vi "Cleanup.vi"(8 "error in":errorcluster, 11 "Refnum In":refnum<vi>) -> (0 "error out":errorcluster)   [LabVIEW 2020, in "FirmataClient.lvlib"]
doc: "Cleanup the library references, data and the actively selected transport (i.e. serial comport)"
uses:
  FirmataClient.lvlib
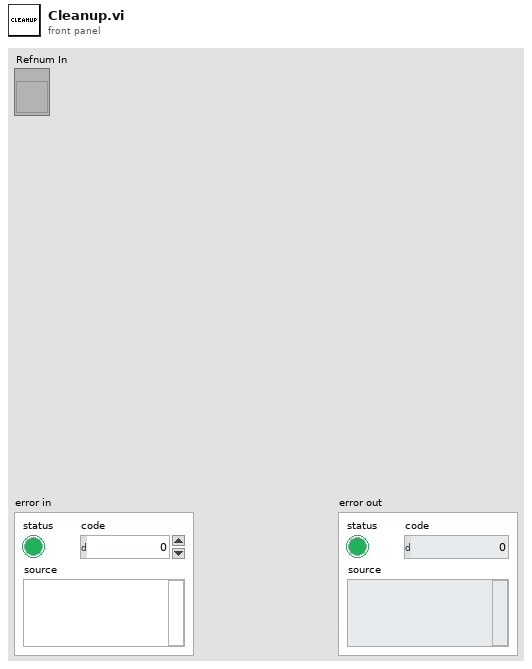
[diagram p1: front panel]
types:
  T1 = typedef "FirmataClient.lvlib/Parameters.ctl" = cluster{"Transport Parameters":T2, "Board Capabilities":map{i32, T4}}
  T2 = typedef "FirmataClient.lvlib/TransportParameters.ctl" = cluster{"Serial Communication":cluster{"Comport":refnum<visa-resource-name>, "No Response Timeout Ms":u32, "Response Complete Timeout Ms":u32, "Max Rx Length":u32, "Baud Rate":u32}, "Selected Transport":T3, "Initializer File Path":path, "Cleaner File Path":path, "Transporter File Path":path}
  T3 = typedef "FirmataClient.lvlib/SupportedTransports.ctl" = enum16{"Serial Communication Port"}
  T4 = typedef "FirmataClient.lvlib/FirmataPinCapabilitiesAndAnalogMapping.ctl" = cluster{"Supported Modes":T5[], "Analog Channel":u8, "Pin Name":string}
  T5 = typedef "FirmataClient.lvlib/FirmataPinCapability.ctl" = cluster{"PinMode":T6, "Resolution":u8}
  T6 = typedef "FirmataClient.lvlib/FirmataPinModes.ctl" = enum16{"DigitalInput", "DigitalOutput", "AnalogInput", "PWM", "Servo", "Shift", "I2C", "OneWire", "Stepper", "Encoder", "Serial", "InputPullup", "Extended.SPI", "Extended.Sonar", "Extended.Tone", "Extended.DHT"}
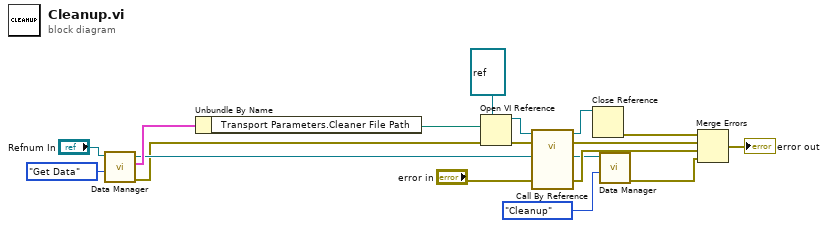
[diagram p0: block diagram]
diagram:
  n1 = call "Data Manager.vi"("Mode"=enum16{"Store Data", "Get Data", "Cleanup"}."Get Data", "Refnum In"="Refnum In") -> ("error out"=w6:errorcluster, "Data Out"=w10:T1, "Refnum Out"=w9:refnum<vi>)  [unwired: 7 in]
  n2 = Unbundle By Name(w10) -> ("Transport Parameters.Cleaner File Path"=w11:path)
  n3 = Open VI Reference(type specifier VI Refnum (for type only)=refnum<vi> refnum, vi path=w11, error in (no error)=w6) -> (vi reference=w16:refnum<vi>, error out=w17:errorcluster)  [unwired: 3 in]
  n4 = call-by-ref "?"(reference=w16, error in=w17, "error in"="error in", "Refnum In"=w9) -> (reference out=w15:refnum<vi>, error out=w14:errorcluster, 0:"error out"=w12:errorcluster, "Refnum Out"=w4:refnum<vi>)  [unwired: 8 in]
  n5 = Close Reference(reference=w15) -> (error out=w13:errorcluster)  [unwired: 1 in]
  n6 = call "Data Manager.vi"("Mode"=enum16{"Store Data", "Get Data", "Cleanup"}."Cleanup", "Refnum In"=w4) -> ("error out"=w3:errorcluster)  [unwired: 7 in, 2 out]
  n7 = Merge Errors(w13, w14, w12, w3) -> (→"error out":errorcluster)
